vi "Basic Level Trigger Detection (obs).vi"   [LabVIEW 2020, in "NI_MAPro.lvlib"]
uses:
  NI_MAPro.lvlib
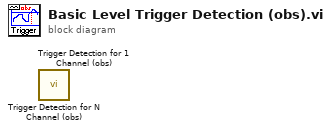
[diagram p0: block diagram]
diagram:
  n1 = call "Trigger Detection for N Channel (obs).vi"() -> ()  [unwired: 13 in, 3 out]
  n2 = call "Trigger Detection for 1 Channel (obs).vi"() -> ()  [unwired: 13 in, 3 out]
